vi "CEIXanes.vi"() -> ()   [LabVIEW 2014]
uses:
  <vilib>/Utility/file.llb/Write To Spreadsheet File (DBL).vi
panel:
  out "Sample Description":string caption="Description"
  out "Zero":bool
  out "Scanning":bool
  out "Moving":bool
  out "min":dbl
  out "max":dbl
  out "Data Saved to:":string
  out "Scan Started":string
  in  "Status":string
  out "Current Sample":string
  in  "ChangeSampleButton":bool
  in  "Select Sample Button":bool
  in  "Current Samples":i32(listbox)
  in  "SelectAnalyzer":bool
  out "error out":errorcluster
  out "Scan Data":cluster{dbl, "element":u32}[](graph)
  in  "ChangeAnalyzerButton":bool
  in  "Current Analyzers":i32(listbox)
  in  "Zero":bool
  in  "eV/step":dbl=1.0
  in  "Low":u32=360
  in  "High":u32=400
  in  "s/sample":dbl=1.0
  in  "Scans":dbl=1.0
  in  "Scan Name":string
  out "Spectrum Graph":dbl[](graph)
  in  "Energy Range":cluster{dbl, dbl}(slide)={0.0, 1.9191919191919191} scale=5090.135010858869..5390.567248588837
  in  "Calibrate":bool
  in  "BeginScan":bool caption="Start Scan"
  in  "Stop":bool
  # "Machine Configuration"
  # "Scan Settings"
  # "Range of Interest"
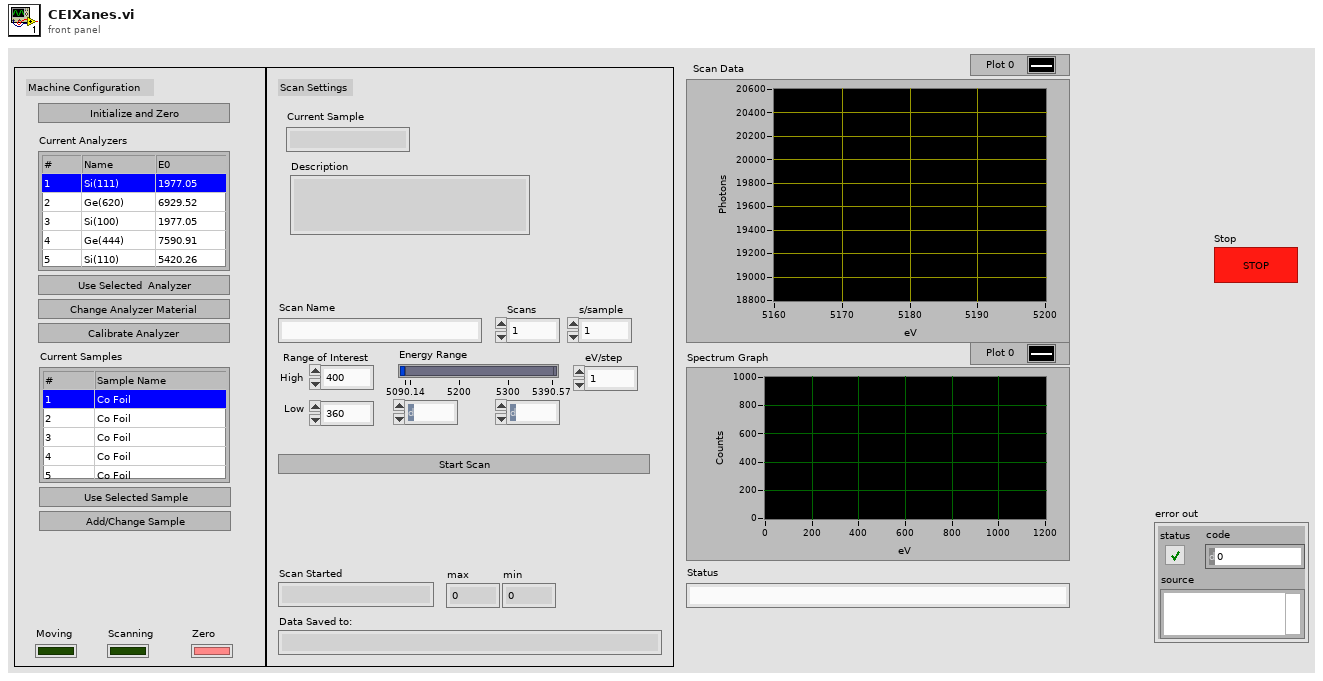
[diagram p1: front panel]
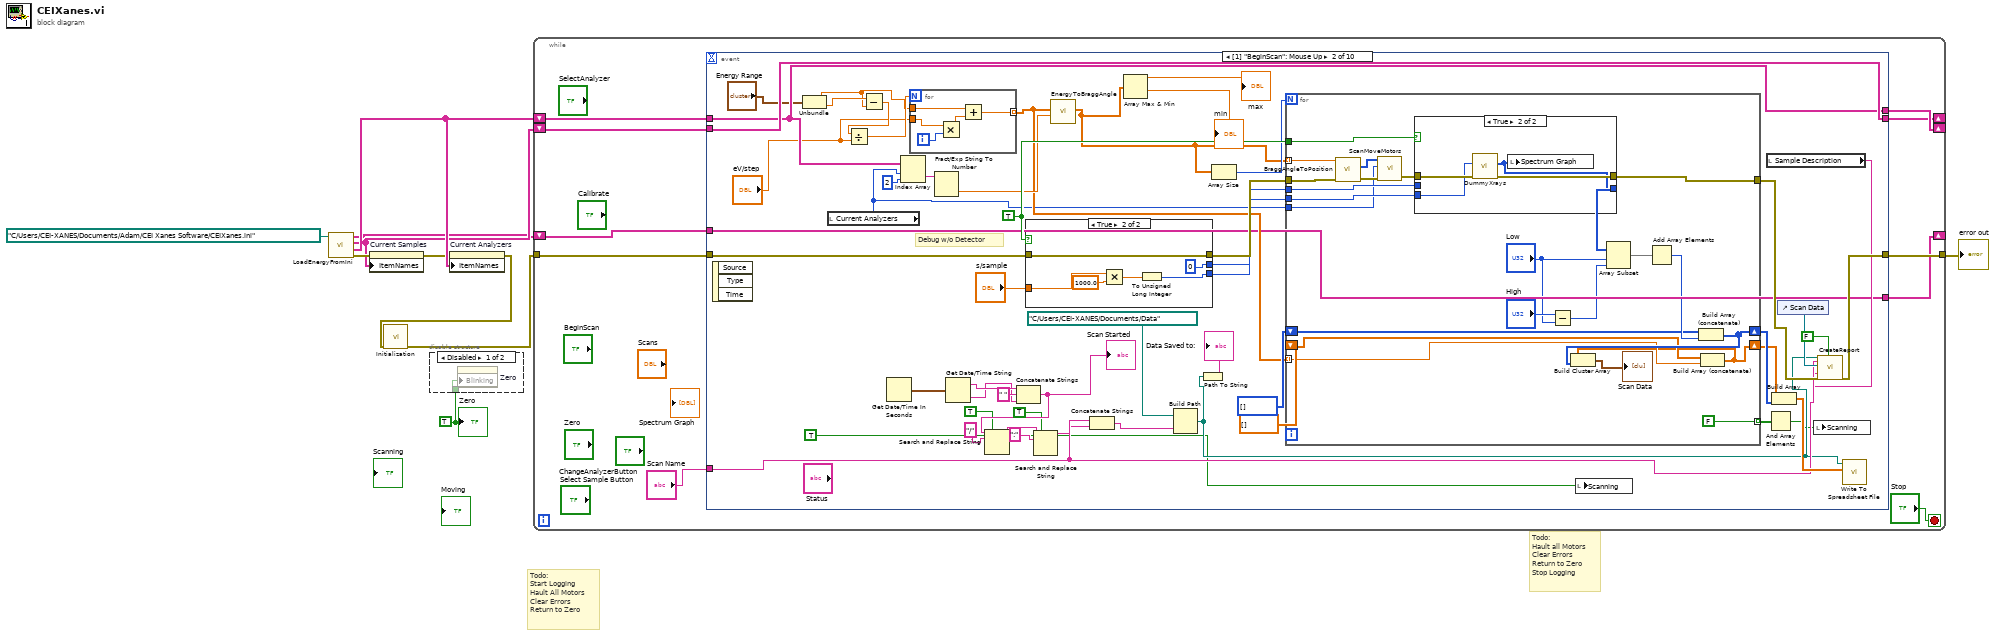
[diagram p0: block diagram]
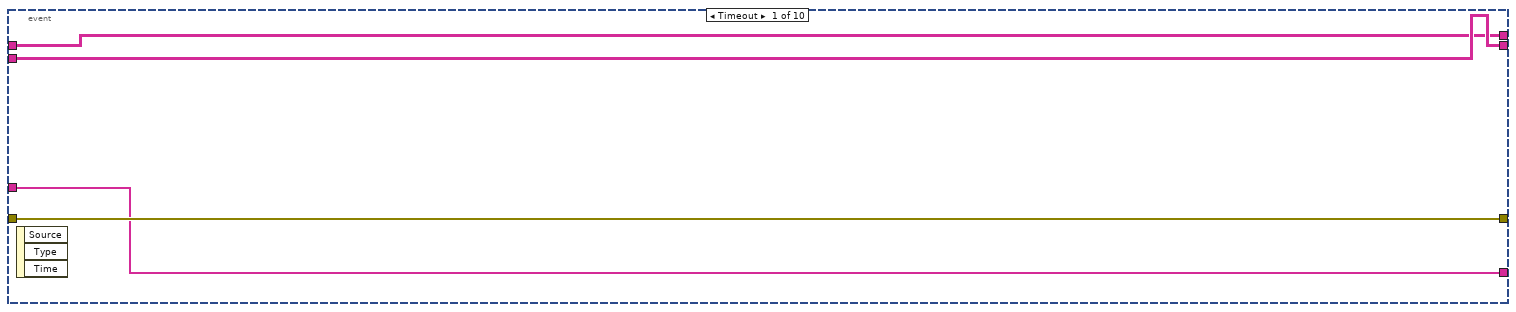
[diagram p3: hidden frame]
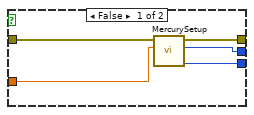
[diagram p4: hidden frame]
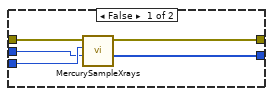
[diagram p5: hidden frame]
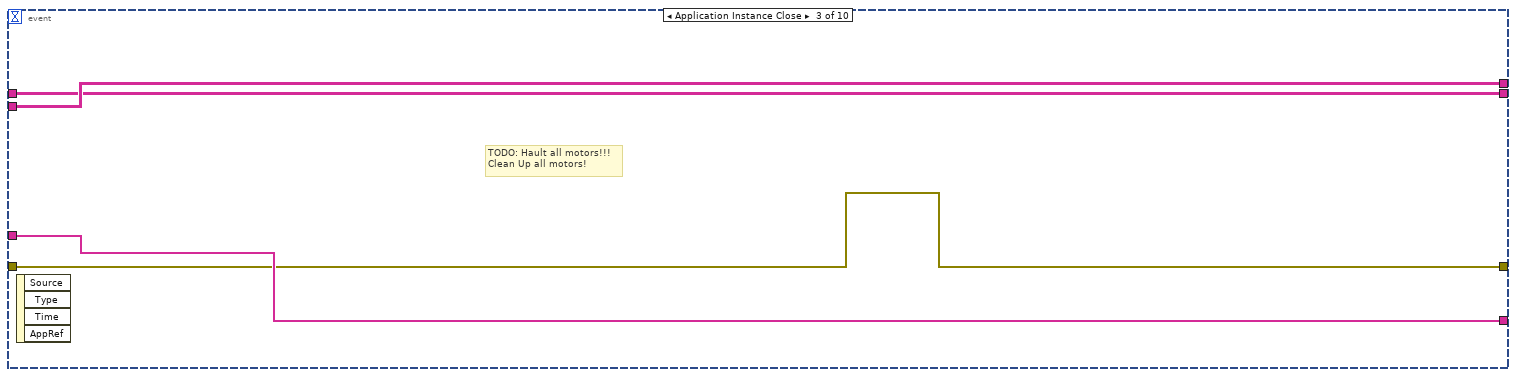
[diagram p6: hidden frame]
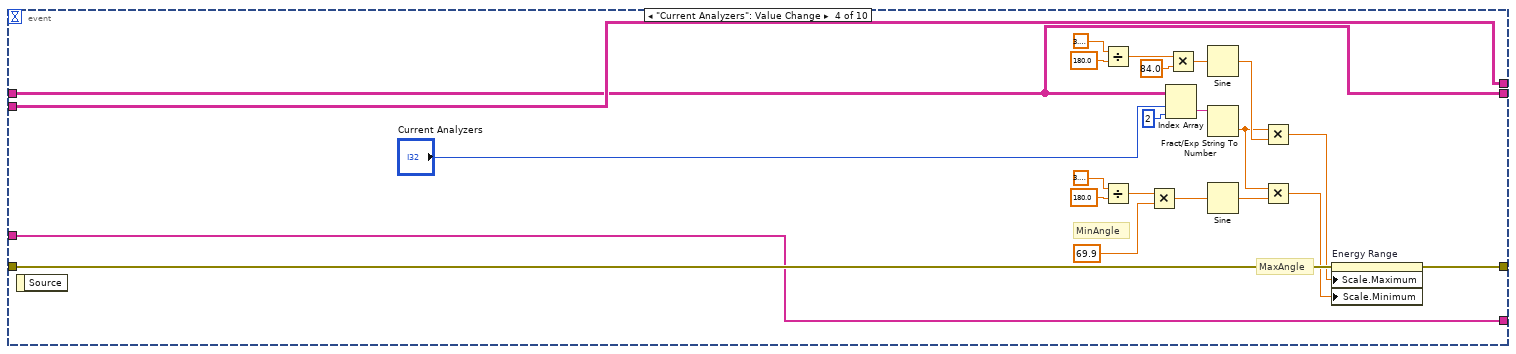
[diagram p7: hidden frame]
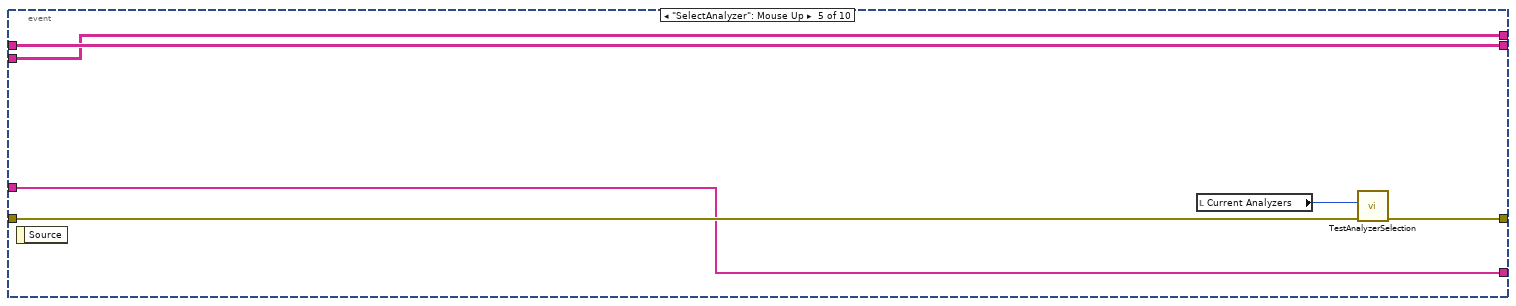
[diagram p8: hidden frame]
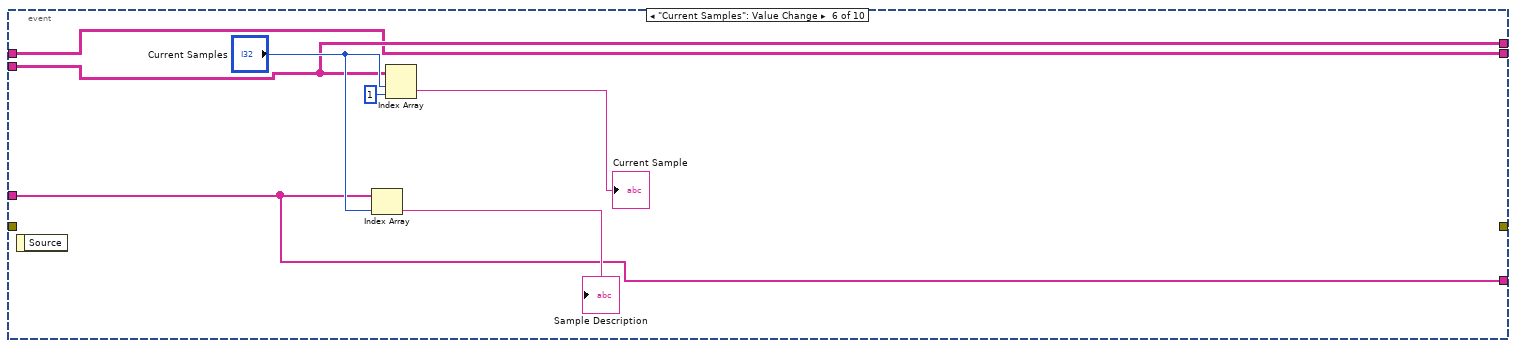
[diagram p9: hidden frame]
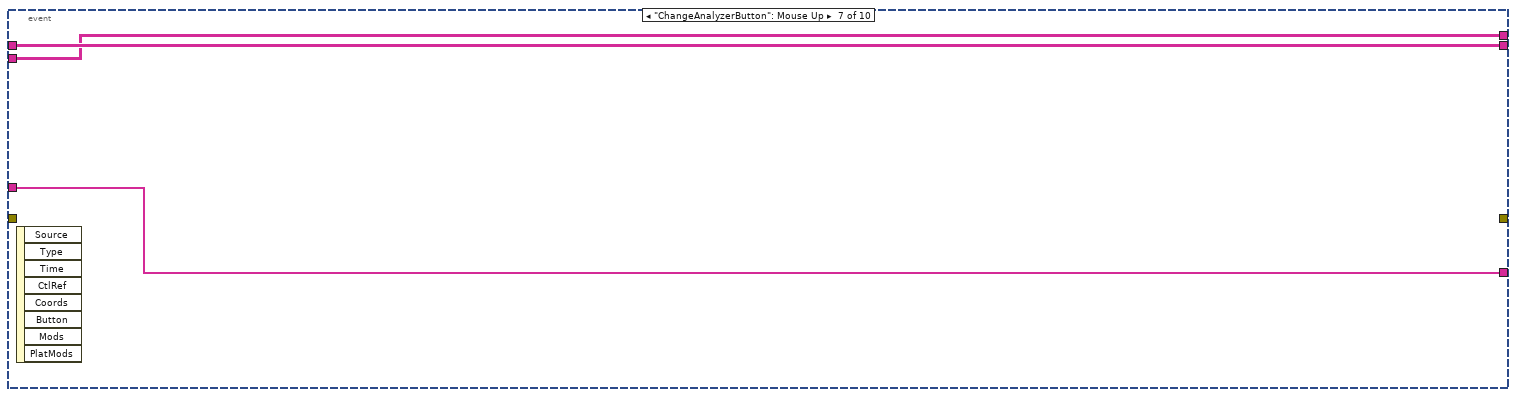
[diagram p10: hidden frame]
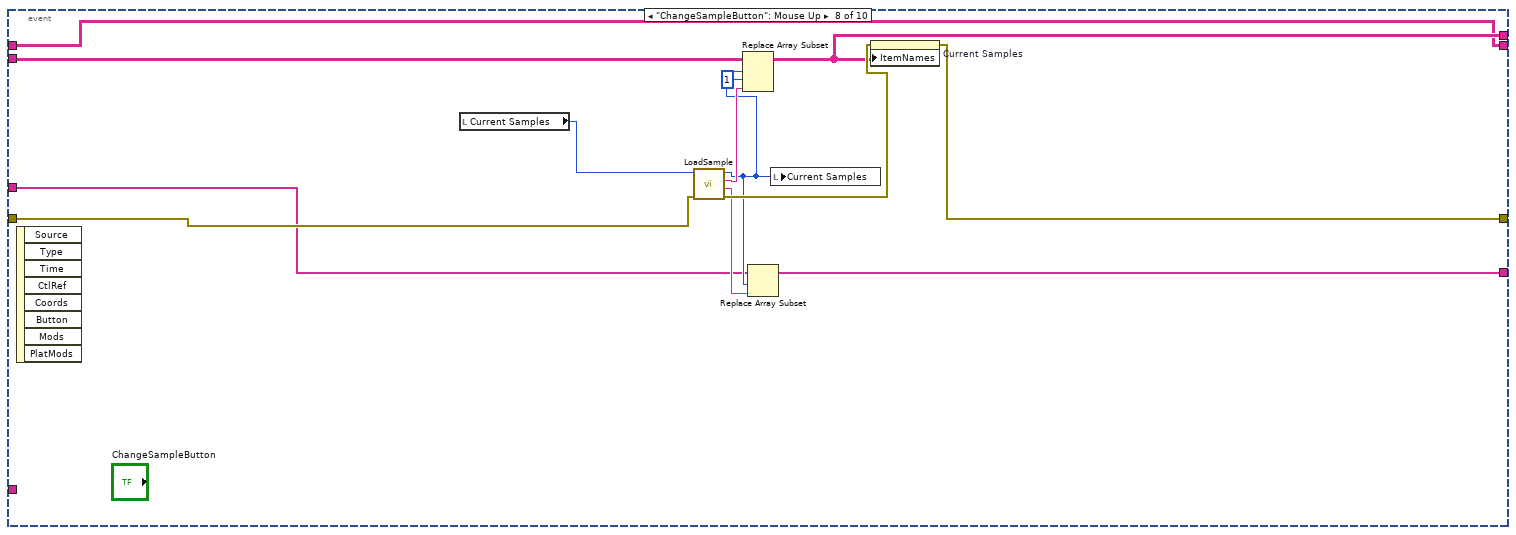
[diagram p11: hidden frame]
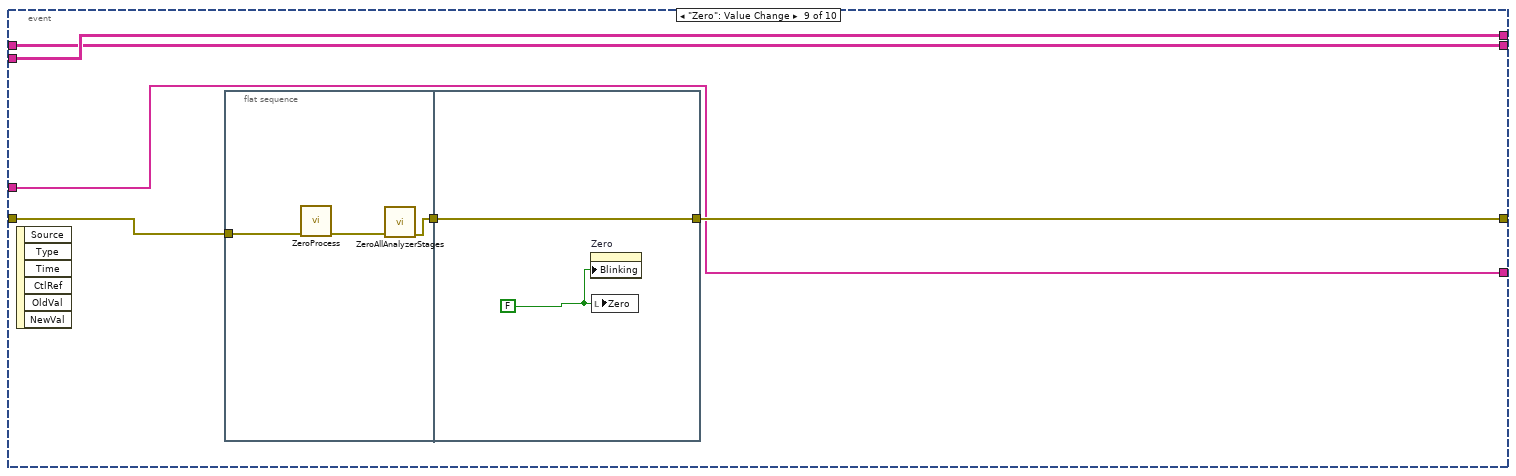
[diagram p12: hidden frame]
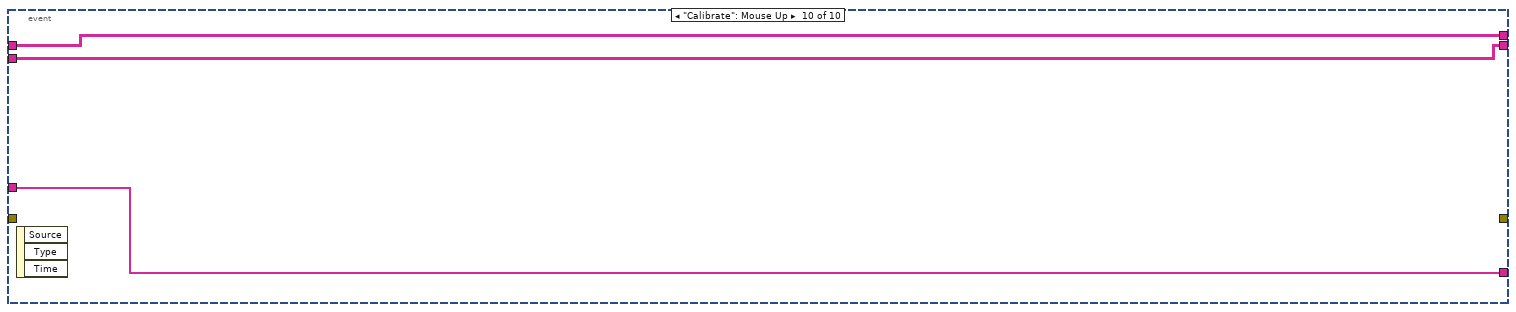
[diagram p13: hidden frame]
diagram:
  w3 = TRUE ("Zero")
  # "Todo:\nHault all Motors\nClear Errors\nReturn to Zero\nStop Logging"
  # "Todo:\nStart Logging\nHault All Motors\nClear Errors\nReturn to Zero"
  n1 = call "LoadEnergyFromIni.vi"("configuration file path"=path "C:/Users/CEI-XANES/Documents/Adam/CEI Xanes Software/CEIXanes.ini") -> ("error out"=w8:errorcluster, "Analyzer Array"=w10:string[][], "Sample Array"=w2:string[][], "SampleDescArray"=w1:string[])  [unwired: 7 in]
  n2 = property on="Current Samples" class="MCListbox (strict)"(error in=w8, "ItemNames"=w2) -> (error out=w7:errorcluster)  [unwired: 1 in, 1 out]
  n3 = disable-structure shown="Disabled" {
    disable-tunnel: w3 -> [w11 _]
    frame Disabled {
      n4 = property on="Zero" class="Bool (strict)"("Blinking"=w11) -> ()  [unwired: 2 in, 2 out]
    }
    frame Enabled {
    }
  }
  n5 = property on="Current Analyzers" class="MCListbox (strict)"(error in=w7, "ItemNames"=w10) -> (error out=w4:errorcluster)  [unwired: 1 in, 1 out]
  n6 = call "Initialization.vi"("error in (no error)"=w4) -> ("error out"=w5:errorcluster)  [unwired: 10 in]
  n7 = while {
    tunnel: w5 -> [w20]
    tunnel: [w19] -> w9
    shift-right: [w12] -> _
    shift-left: w10 -> [w18]
    shift-right: [w13] -> _
    shift-left: w1 -> [w15]
    shift-right: [w14] -> _
    shift-left: w2 -> [w16]
    stop <- "Stop" stop-if-true
    n8 = event shown="[1] \"BeginScan\": Mouse Up" {
      selector: _ -> [_ _ _ _ _ _ _ _ _ _]
      dyn-events: _ -> [_ _ _ _ _ _ _ _ _ _]
      timeout: _ -> [_ _ _ _ _ _ _ _ _ _]
      tunnel: w20 -> [w25 w77 w127 w141 w158 _ _ w182 w188 _]
      tunnel: [w25 w55 w127 w139 w157 _ _ w176 w187 _] -> w19
      tunnel: w18 -> [w23 w29 w128 w131 w155 w160 w169 w170 w183 w194]
      tunnel: "Scan Name" -> [_ w52 _ _ _ _ _ _ _ _]
      tunnel: w16 -> [w24 w30 w129 w132 w154 w161 w167 w180 w184 w195]
      tunnel: w15 -> [w22 w28 w130 w133 w156 w162 w168 w173 w185 w196]
      tunnel: [w23 w29 w129 w132 w154 w161 w167 w172 w184 w194] -> w14
      tunnel: [w22 w28 w130 w133 w156 w162 w168 w171 w185 w196] -> w13
      tunnel: [w24 w30 w128 w131 w155 w160 w169 w170 w183 w195] -> w12
      event Timeout {
        n9 = event-data() -> ()  [unwired: 1 in, 3 out]
      }
      event "BeginScan": Mouse Up {
        w78 = TRUE
        # "Debug w/o Detector"
        n10 = event-data() -> ()  [unwired: 1 in, 3 out]
        n11 = Unbundle("Energy Range") -> (w67:dbl, w70:dbl)
        n12 = local read "Current Analyzers"() -> (w61:i32)
        n13 = Subtract(x=w70, y=w67) -> (x-y=w69:dbl)
        n14 = Divide(x=w69, y="eV/step") -> (x/y=w68:dbl)
        n15 = Get Date/Time In Seconds() -> (seconds since 1Jan1904=w45:timestamp)
        n16 = Index Array(array=w29, index (row)=w61, index (col)=2 ("disabled index (col)")) -> (element=w65:string)
        n17 = for {
          N: w68 -> [_]
          tunnel: "eV/step" -> [w81]
          tunnel: w67 -> [w83]
          tunnel: [w79] -> w63 mode=indexing
          i -> [w82]
          n18 = Multiply(x=w81, y=w82) -> (x*y=w80:dbl)
          n19 = Add(x=w83, y=w80) -> (x+y=w79:dbl)
        }
        n20 = Fract/Exp String To Number(string=w65) -> (number=w64:dbl)  [unwired: 3 in, 1 out]
        n21 = Get Date/Time String(seconds (now)=w45) -> (date string=w53:string, time string=w43:string)  [unwired: 2 in]
        n22 = Concatenate Strings(w53, " " ("string"), w43) -> (w41:string)
        "Scan Started" <- w41
        n23 = Search and Replace String(replace all?=TRUE ("replace all? (F)"), input string=w41, search string="/" ("substring (\"\")")) -> (result string=w40:string)  [unwired: 5 in, 3 out]
        n24 = case shown="True" w78 {
          tunnel: w77 -> [w88 w90]
          tunnel: [w87 w90] -> w76
          tunnel: "s/sample" -> [w86 w94]
          tunnel: [w85 w92] -> w74
          tunnel: [w84 0 ("detChan")] -> w73
          frame False {
            n25 = call "MercurySetup.vi"("error in (no error)"=w88, "CollectionTime"=w86) -> ("error out"=w87:errorcluster, "detChan"=w84:i32, "CollectionTime"=w85:u32)  [unwired: 4 in, 2 out]
          }
          frame True {
            n26 = Multiply(x=w94, y=1000.0) -> (x*y=w91:dbl)
            n27 = To Unsigned Long Integer(number=w91) -> (unsigned 32bit integer=w92:u32)
          }
        }
        n28 = Search and Replace String(replace all?=TRUE ("replace all? (F)"), input string=w40, search string=":" ("substring (\"\")")) -> (result string=w42:string)  [unwired: 5 in, 3 out]
        n29 = call "EnergyToBraggAngle.vi"("E0"=w64, "EnergyIn"=w63) -> ("BraggOut"=w48:dbl[])  [unwired: 9 in]
        n30 = Concatenate Strings(w52, w42) -> (w51:string)
        n31 = Array Max & Min(array=w48) -> (max value=→"max":dbl, min value=→"min":dbl)  [unwired: 2 out]
        n32 = Build Path(base path=path "C:/Users/CEI-XANES/Documents/Data", name or relative path=w51) -> (appended path=w35:path)
        n33 = Path To String(path=w35) -> (string=→"Data Saved to:":string)
        n34 = Array Size(array=w48) -> (size(s)=w71:i32)
        n35 = for {
          N: w71 -> [_]
          tunnel: w78 -> [w117]
          tunnel: w76 -> [w116]
          tunnel: w74 -> [w115]
          tunnel: [w114] -> w56
          tunnel: w73 -> [w113]
          shift-right: [w104] -> w60
          shift-left: u32[] [] -> [w106]
          tunnel: w48 -> [w105] mode=indexing
          tunnel: w63 -> [w102] mode=indexing
          shift-right: [w100] -> w59
          shift-left: dbl[] [] -> [w101]
          tunnel: w61 -> [w95]
          tunnel: [FALSE] -> w33 mode=indexing
          n36 = call "BraggAngleToPosition.vi"("Error In"=w116, "BraggAngle"=w105) -> ("Error Out"=w97:errorcluster, "appended array"=w96:i32[])  [unwired: 8 in]
          n37 = call "ScanMoveMotors.vi"("error constant"=w97, "AnalyzerNumber"=w95, "PulseArrayIn"=w96) -> ("error constant 2"=w98:errorcluster)  [unwired: 8 in]
          n38 = case shown="True" w117 {
            tunnel: w98 -> [w122 w126]
            tunnel: [w121 w125] -> w114
            tunnel: w115 -> [w120 w124]
            tunnel: [w119 w123] -> w112
            tunnel: w113 -> [w118 _]
            frame False {
              n39 = call "MercurySampleXrays.vi"("detChan"=w118, "Collection Time"=w120, "error in (no error)"=w122) -> ("SpectrumData"=w119:i32[], "error out"=w121:errorcluster)  [unwired: 7 in]
            }
            frame True {
              n40 = call "DummyXrays.vi"("error in"=w126, "Delay"=w124) -> ("error out"=w125:errorcluster, "DummySpectrum"=w123:u32[])  [unwired: 8 in]
              n41 = local write "Spectrum Graph"(w123) -> ()
            }
          }
          n42 = Subtract(x="High", y="Low") -> (x-y=w111:u32)
          n43 = Array Subset(array=w112, index="Low", length=w111) -> (w108:u32[])
          n44 = Add Array Elements(numeric array=w108) -> (sum=w107:u32)
          n45 = Build Array (concatenate)(w106, w107) -> (w104:u32[])
          n46 = Build Array (concatenate)(w101, w102) -> (w100:dbl[])
          n47 = Build Cluster Array(w100, w104) -> (→"Scan Data":cluster{dbl, "element":u32}[])
        }
        n48 = local write "Scanning"(TRUE ("Scanning")) -> ()
        n49 = local read "Sample Description"() -> (w31:string)
        n50 = And Array Elements(Boolean array=w33) -> (logical AND=w32:bool)
        n51 = Build Array(w59, w60) -> (w54:dbl[][])
        n52 = control-ref of="Scan Data"() -> (w58:refnum<vi>)
        n53 = local write "Scanning"(w32) -> ()
        n54 = call "CreateReport.vi"("ReportName"=w35, "SampleName"=w52, "ctrl reference"=w58, "Sample Desription"=w31, "error in (no error)"=w56, "PrintReport"=FALSE) -> ("error out"=w55:errorcluster)  [unwired: 13 in]
        n55 = call-poly <vilib>:"Write To Spreadsheet File.vi"("2D data"=w54, "file path (dialog if empty)"=w35) -> ()  [unwired: 6 in, 1 out]
      }
      event Application Instance Close {
        # "TODO: Hault all motors!!!\nClean Up all motors!"
        n56 = event-data() -> ()  [unwired: 1 in, 4 out]
      }
      event "Current Analyzers": Value Change {
        # "MaxAngle"
        # "MinAngle"
        n57 = event-data() -> ()  [unwired: 1 in, 1 out]
        n58 = Divide(x=3.141592653589793, y=180.0) -> (x/y=w151:dbl)
        n59 = Divide(x=3.141592653589793, y=180.0) -> (x/y=w146:dbl)
        n60 = Multiply(x=w146, y=69.9) -> (x*y=w142:dbl)
        n61 = Index Array(array=w131, index (row)="Current Analyzers", index (col)=2 ("disabled index (col)")) -> (element=w136:string)
        n62 = Multiply(x=w151, y=84.0) -> (x*y=w150:dbl)
        n63 = Sine(x=w150) -> (sin(x)=w143:dbl)
        n64 = Fract/Exp String To Number(string=w136) -> (number=w135:dbl)  [unwired: 3 in, 1 out]
        n65 = Sine(x=w142) -> (sin(x)=w144:dbl)
        n66 = Multiply(x=w135, y=w143) -> (x*y=w140:dbl)
        n67 = Multiply(x=w135, y=w144) -> (x*y=w138:dbl)
        n68 = property on="Energy Range" class="Slide (strict)"(error in=w141, "Scale.Maximum"=w140, "Scale.Minimum"=w138) -> (error out=w139:errorcluster)  [unwired: 1 in, 1 out]
      }
      event "SelectAnalyzer": Mouse Up {
        n69 = event-data() -> ()  [unwired: 1 in, 1 out]
        n70 = local read "Current Analyzers"() -> (w159:i32)
        n71 = call "TestAnalyzerSelection.vi"("error in"=w158, "Analyzer"=w159) -> ("error out"=w157:errorcluster)  [unwired: 9 in]
      }
      event "Current Samples": Value Change {
        n72 = event-data() -> ()  [unwired: 1 in, 1 out]
        n73 = Index Array(array=w162, index="Current Samples") -> (element=→"Sample Description":string)
        n74 = Index Array(array=w161, index (row)="Current Samples", index (col)=1 ("disabled index (col)")) -> (element=→"Current Sample":string)
      }
      event "ChangeAnalyzerButton": Mouse Up {
        n75 = event-data() -> ()  [unwired: 1 in, 8 out]
      }
      event "ChangeSampleButton": Mouse Up {
        n76 = event-data() -> ()  [unwired: 1 in, 8 out]
        n77 = local read "Current Samples"() -> (w181:i32)
        n78 = call "LoadSample.vi"("error constant"=w182, "SampleNumberToLoad"=w181) -> ("error out"=w177:errorcluster, "Sample Details 2"=w175:string, "Name of Sample 2"=w179:string, "CurrentSample"=w174:i32)  [unwired: 6 in]
        n79 = Replace Array Subset(array=w180, new element=w179, index (row)=w174, index (col)=1 ("disabled index (col)")) -> (w172:string[][])
        n80 = Replace Array Subset(array=w173, new element=w175, index=w174) -> (w171:string[])
        n81 = local write "Current Samples"(w174) -> ()
        n82 = property on="Current Samples" class="MCListbox (strict)"(error in=w177, "ItemNames"=w172) -> (error out=w176:errorcluster)  [unwired: 1 in, 1 out]
      }
      event "Zero": Value Change {
        n83 = event-data() -> ()  [unwired: 1 in, 6 out]
        n84 = flat-sequence {
          tunnel: w188 -> [w191]
          tunnel: [w189] -> w186
          tunnel: [w193] -> w187
          tunnel: w186 -> [w193]
          frame #0 {
            n85 = call "ZeroProcess.vi"("error in (no error)"=w191) -> ("error out"=w190:errorcluster)  [unwired: 10 in]
            n86 = call "ZeroAllAnalyzerStages.vi"("error in (no error)"=w190) -> ("error out"=w189:errorcluster)  [unwired: 10 in]
          }
          frame #1 {
            w192 = FALSE ("Zero")
            n87 = property on="Zero" class="Bool (strict)"("Blinking"=w192) -> ()  [unwired: 2 in, 2 out]
            n88 = local write "Zero"(w192) -> ()
          }
        }
      }
      event "Calibrate": Mouse Up {
        n89 = event-data() -> ()  [unwired: 1 in, 3 out]
      }
    }
  }
  "error out" <- w9
  "Zero" <- w3
